vi "Configure Aperture_.vi"(5 "Measurement Time (1: Medium)":u16(ring)=1 items=["Short", "Medium", "Long"], 7 "Averaging Factor (1)":i32=1, 8 "error in (no error)":errorcluster, 11 "Agilent E4980 in":refnum<class "Agilent E4980.lvclass">) -> (0 "error out":errorcluster, 3 "Agilent E4980 out":refnum<class "Agilent E4980.lvclass">)   [LabVIEW 2020, in "Agilent E4980.lvclass"]
uses:
  Agilent E4980.lvclass
  C:/Sandbox/RF Bench/Source Code/WiSpry Test Framework/Instruments/Instrument.lvclass
  Instrument.lvclass/Instrument.ctl
  Instrument.lvclass
  <instrlib>/Agilent E4980/Agilent E4980.lvlib
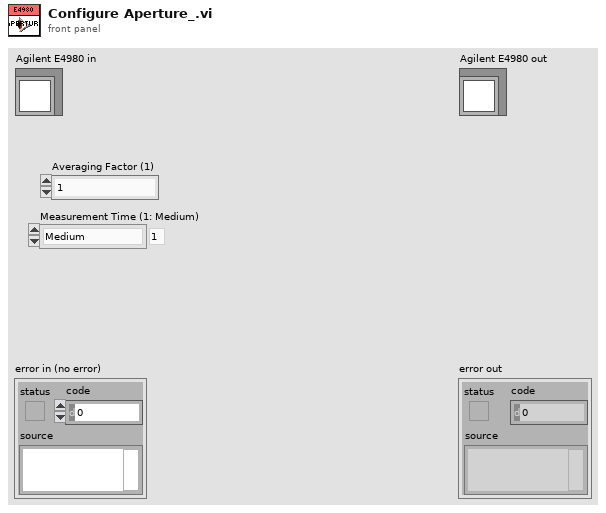
[diagram p1: front panel]
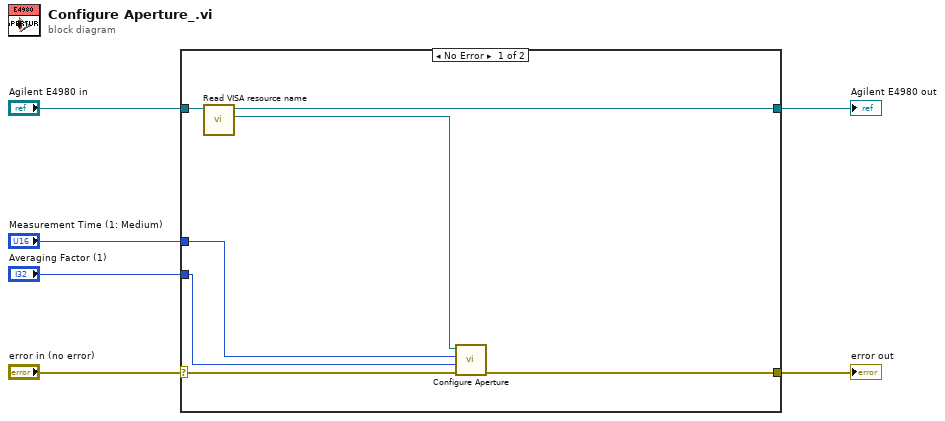
[diagram p0: block diagram]
diagram:
  n1 = case shown="No Error" "error in (no error)" {
    selector: "error in (no error)" -> [w10 w15]
    tunnel: [w9 w15] -> w1
    tunnel: [w12 w14] -> w5
    tunnel: "Agilent E4980 in" -> [w13 w14]
    tunnel: "Measurement Time (1: Medium)" -> [w8 _]
    tunnel: "Averaging Factor (1)" -> [w7 _]
    frame No Error {
      n2 = call "Read VISA resource name.vi"("Instrument in"=w13) -> ("VISA resource name"=w11:refnum<visa-resource-name>, "Instrument out"=w12:refnum<class "Agilent E4980.lvclass">)  [unwired: 9 in]
      n3 = call <instrlib>:"Configure Aperture.vi"("error in (no error)"=w10, "Averaging Factor (1)"=w7, "Measurement Time (1: Medium)"=w8, "VISA resource name"=w11) -> ("error out"=w9:errorcluster)  [unwired: 6 in, 1 out]
    }
    frame Error {
    }
  }
  "error out" <- w1
  "Agilent E4980 out" <- w5
